vi "create_black_screen.vi"() -> (1 "img_black_screen":T1(plugin-control))   [LabVIEW 2011]
uses:
  global_vars.vi
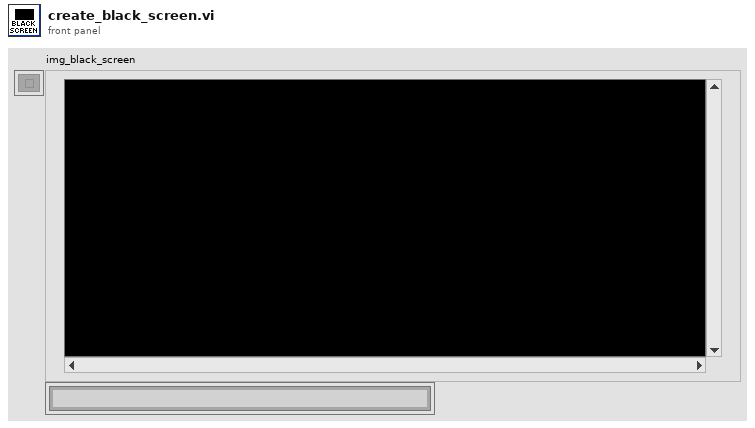
[diagram p1: front panel]
types:
  T1 = typedef "IMAQ Image.ctl" = refnum<image>
  T2 = typedef "Image Type" = u32
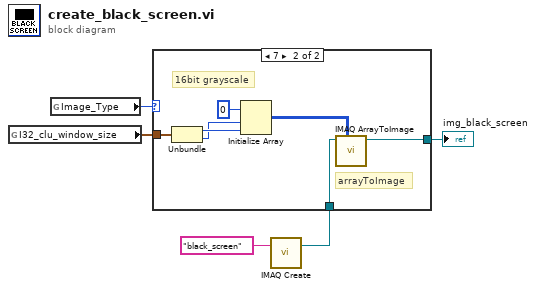
[diagram p0: block diagram]
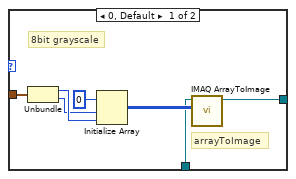
[diagram p2: hidden frame]
diagram:
  n1 = global read "global_vars.vi" "I32_clu_window_size"() -> (w3:cluster{"x Width(Px)":i32, "y height(Px)":i32})
  n2 = global read "global_vars.vi" "Image_Type"() -> (w5:T2)
  n3 = call "IMAQ Create"("Image Name"="black_screen") -> ("New Image"=w1:T1)  [unwired: 3 in, 2 out]
  n4 = case shown="7" w5 {
    tunnel: [w8 w16] -> w4
    tunnel: w3 -> [w7 w14]
    tunnel: w1 -> [w6 w13]
    frame 0, Default {
      # "8bit grayscale"
      # "arrayToImage"
      n5 = Unbundle(w7) -> ("x Width(Px)"=w12:i32, "y height(Px)"=w11:i32)
      n6 = Initialize Array(u8 0 ("element"), w11, w12) -> (w9:u8[][])
      n7 = call "IMAQ ArrayToImage"("Image Pixels (U8)"=w9, "Image"=w6) -> ("Image Out"=w8:T1)  [unwired: 8 in, 1 out]
    }
    frame 7 {
      # "16bit grayscale"
      # "arrayToImage"
      n8 = Unbundle(w14) -> ("x Width(Px)"=w19:i32, "y height(Px)"=w18:i32)
      n9 = Initialize Array(u16 0 ("element"), w18, w19) -> (w15:u16[][])
      n10 = call "IMAQ ArrayToImage"("Image Pixels (U16)"=w15, "Image"=w13) -> ("Image Out"=w16:T1)  [unwired: 8 in, 1 out]
    }
  }
  "img_black_screen" <- w4
